vi "Select Standard Sheet.vi"(8 "error in (no error)":errorcluster, 11 "Excel Logger in":refnum<class "Excel Logger.lvclass">) -> (0 "error out":errorcluster, 3 "Excel Logger out":refnum<class "Excel Logger.lvclass">)   [LabVIEW 2014, in "Excel Logger.lvclass"]
uses:
  Excel Logger.lvclass
  Excel Logger.lvclass/Excel Logger.ctl
  Data Analyser Report/Data Analyser Report.lvclass
  Excel Interface/Excel Interface.lvclass
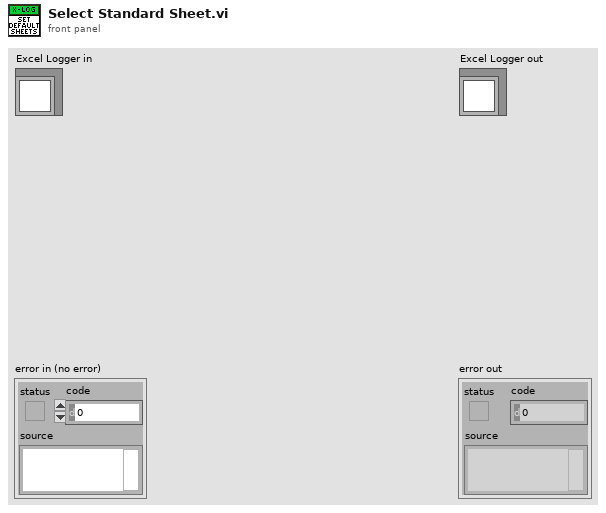
[diagram p1: front panel]
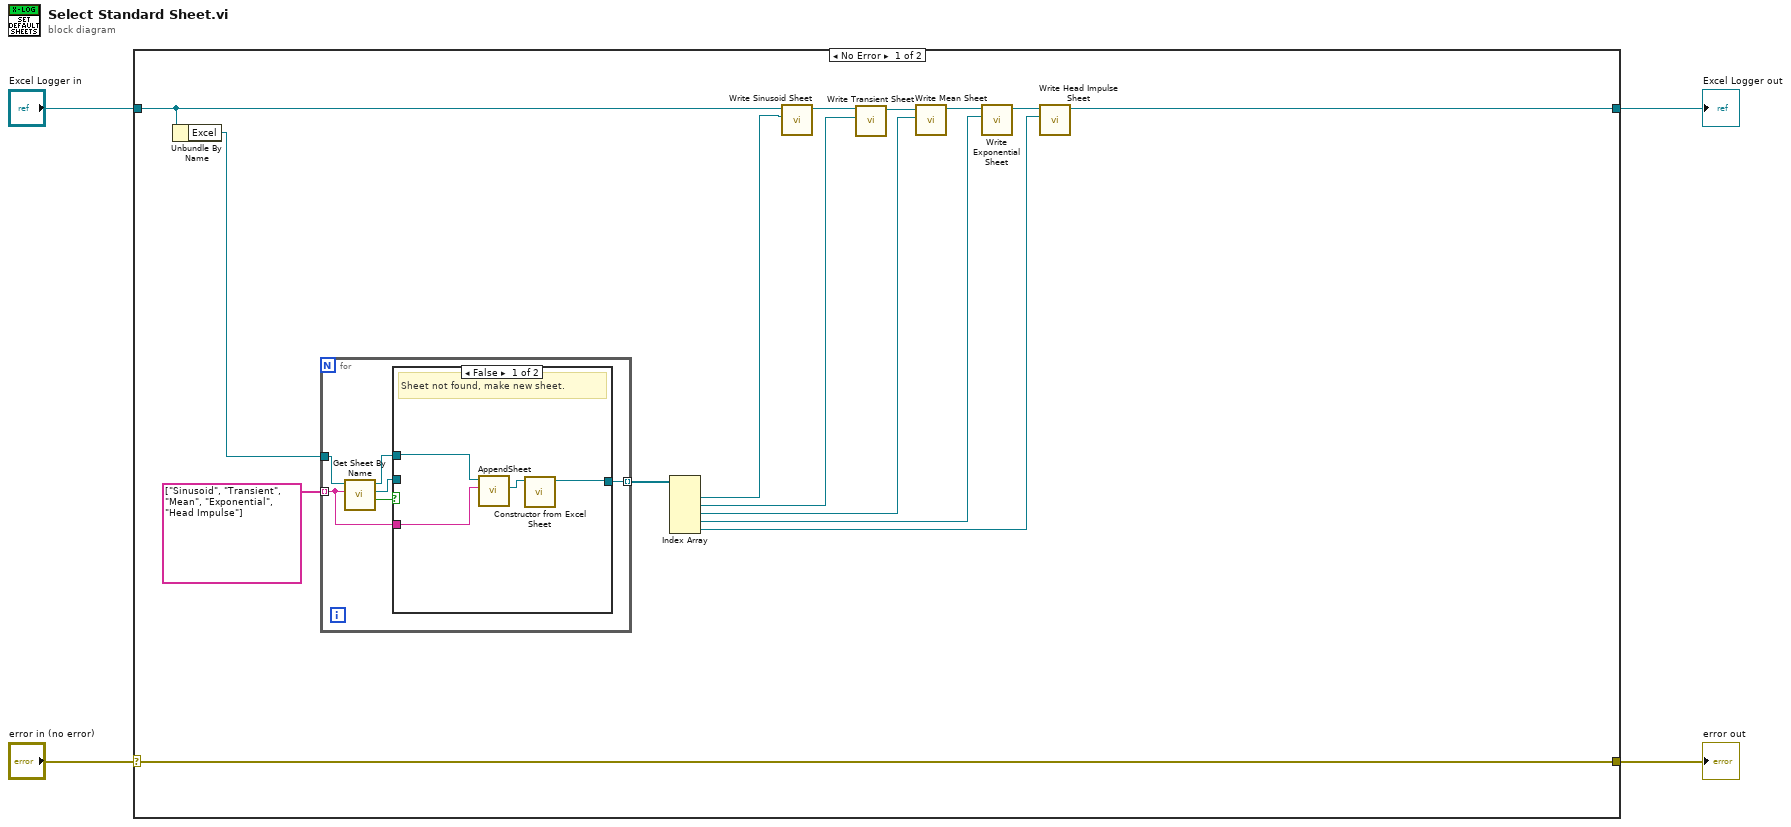
[diagram p0: block diagram]
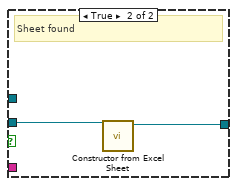
[diagram p2: hidden frame]
diagram:
  n1 = case shown="No Error" "error in (no error)" {
    selector: "error in (no error)" -> [w19 w33]
    tunnel: [w19 w33] -> w3
    tunnel: [w6 w32] -> w1
    tunnel: "Excel Logger in" -> [w18 w32]
    frame No Error {
      n2 = Unbundle By Name(w18) -> ("Excel"=w13:refnum<class "Excel Interface.lvclass">)
      n3 = for {
        tunnel: string[] ["Sinusoid", "Transient", "Mean", "Exponential", "Head Impulse"] -> [w20] mode=indexing
        tunnel: w13 -> [w23]
        tunnel: [w22] -> w12 mode=indexing
        n4 = call "Get Sheet By Name.vi"("Name"=w20, "Excel Interface in"=w23) -> ("Sheet Found?"=w25:bool, "Excel Sheet out"=w24:refnum<class "Excel Sheet.lvclass">, "Excel Interface out"=w21:refnum<class "Excel Interface.lvclass">)  [unwired: 6 in, 1 out]
        n5 = case shown="False" w25 {
          tunnel: w24 -> [_ w31]
          tunnel: [w26 w30] -> w22
          tunnel: w21 -> [w28 _]
          tunnel: w20 -> [w27 _]
          frame False {
            # "Sheet not found, make new sheet."
            n6 = call "AppendSheet.vi"("Name"=w27, "Excel Interface in"=w28) -> ("Excel Sheet out"=w29:refnum<class "Excel Sheet.lvclass">)  [unwired: 7 in, 2 out]
            n7 = call "Constructor from Excel Sheet.vi"("Excel Sheet.lvclass"=w29) -> ("Data Analyser Report.lvclass"=w26:refnum<class "Data Analyser Report.lvclass">)  [unwired: 10 in]
          }
          frame True {
            # "Sheet found"
            n8 = call "Constructor from Excel Sheet.vi"("Excel Sheet.lvclass"=w31) -> ("Data Analyser Report.lvclass"=w30:refnum<class "Data Analyser Report.lvclass">)  [unwired: 10 in]
          }
        }
      }
      n9 = Index Array(array=w12) -> (element #1=w11:refnum<class "Data Analyser Report.lvclass">, element #2=w10:refnum<class "Data Analyser Report.lvclass">, element #3=w9:refnum<class "Data Analyser Report.lvclass">, element #4=w8:refnum<class "Data Analyser Report.lvclass">, element #5=w5:refnum<class "Data Analyser Report.lvclass">)  [unwired: 5 in]
      n10 = call "Write Sinusoid Sheet.vi"("Data Analyser Report.lvclass"=w11, "Excel Logger in"=w18) -> ("Excel Logger out"=w17:refnum<class "Excel Logger.lvclass">)  [unwired: 8 in, 1 out]
      n11 = call "Write Transient Sheet.vi"("Data Analyser Report.lvclass"=w10, "Excel Logger in"=w17) -> ("Excel Logger out"=w16:refnum<class "Excel Logger.lvclass">)  [unwired: 8 in, 1 out]
      n12 = call "Write Mean Sheet.vi"("Data Analyser Report.lvclass"=w9, "Excel Logger in"=w16) -> ("Excel Logger out"=w15:refnum<class "Excel Logger.lvclass">)  [unwired: 8 in, 1 out]
      n13 = call "Write Exponential Sheet.vi"("Exponential"=w8, "Excel Logger in"=w15) -> ("Excel Logger out"=w7:refnum<class "Excel Logger.lvclass">)  [unwired: 8 in, 1 out]
      n14 = call "Write Head Impulse Sheet.vi"("Head Impulse"=w5, "Excel Logger in"=w7) -> ("Excel Logger out"=w6:refnum<class "Excel Logger.lvclass">)  [unwired: 8 in, 1 out]
    }
    frame Error {
    }
  }
  "error out" <- w3
  "Excel Logger out" <- w1
